vi "Create Data File.vi"(8 "Error In":errorcluster) -> (0 "Error Out":errorcluster, 3 "File Refnum":refnum<file>)   [LabVIEW 2014]
doc: "This VI performs a series of tasks to create a file for logging data:\n\n1) Check to see if a folder called 'Logged Data' exsists in the same directory as the application\n2) If the folder does not exsist, create it\n3) Create a file name of the format 'Acquired Data <Date> <Time>.txt'\n4) Replace or Create the file"
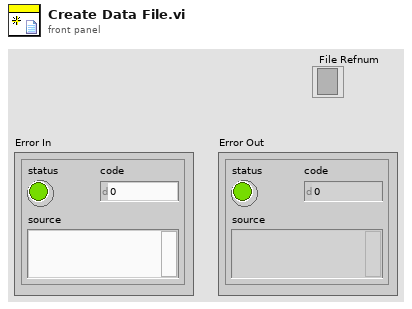
[diagram p1: front panel]
types:
  T1 = enum16{"open", "replace", "create", "open or create", "replace or create", "replace or create with confirmation"}
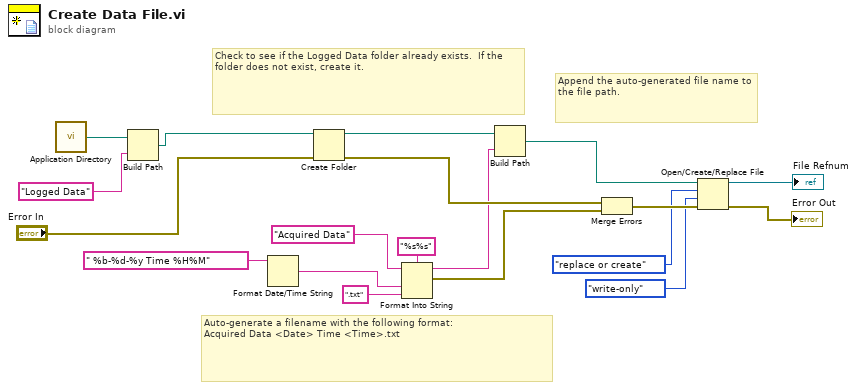
[diagram p0: block diagram]
diagram:
  # "Append the auto-generated file name to the file path."
  # "Check to see if the Logged Data folder already exists.  If the folder does not exist, create it."
  # "Auto-generate a filename with the following format:\nAcquired Data <Date> Time <Time>.txt"
  n1 = call <vilib>:"Application Directory.vi"() -> ("Application Directory"=w10:path)
  n2 = Build Path(base path=w10, name or relative path="Logged Data" ("prompt (Create Folder)")) -> (appended path=w2:path)
  n3 = Format Date/Time String(time format string (%c)=" %b-%d-%y Time %H%M") -> (date/time string=w6:string)  [unwired: 2 in]
  n4 = Create Folder(path (use dialog)=w2, error in="Error In") -> (created path=w13:path, error out=w12:errorcluster)  [unwired: 1 in, 1 out]
  n5 = Format Into String(format string="%s%s", initial string="Acquired Data" ("string"), w6, ".txt" ("string")) -> (resulting string=w3:string, error out=w4:errorcluster)  [unwired: 1 in]
  n6 = Build Path(base path=w13, name or relative path=w3) -> (appended path=w19:path)
  n7 = Merge Errors(w12, w4) -> (w18:errorcluster)
  n8 = Open/Create/Replace File(file path (use dialog)=w19, error in=w18, operation (0:open)=T1."replace or create", access (0:read/write)=enum16{"read/write", "read-only", "write-only"}."write-only") -> (refnum out=→"File Refnum":refnum<file>, error out=→"Error Out":errorcluster)  [unwired: 2 in, 1 out]
